vi "Change detector with tolerance threshold-DBL.vi"(6 "Tolerance (0.000001)":dbl=1e-06 format="%#_13f", 9 "From file":dbl[](array[numeric]), 11 "Current values":dbl[](array[numeric])) -> (2 "Changed?":bool[](array[boolean]))   [LabVIEW 2017]
panel:
  out "Difference":dbl[](array[numeric]) format="%#_6f"
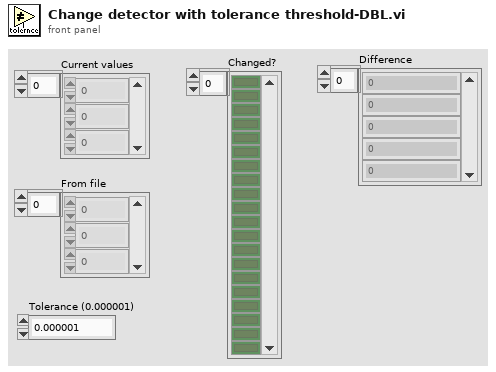
[diagram p1: front panel]
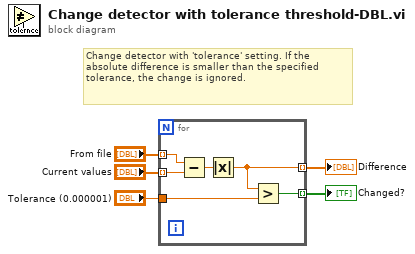
[diagram p0: block diagram]
diagram:
  # "Change detector with 'tolerance' setting. If the absolute difference is smaller than the specified tolerance, the change is ignored."
  n1 = for {
    tunnel: "From file" -> [w11] mode=indexing
    tunnel: "Current values" -> [w10] mode=indexing
    tunnel: [w6] -> w3 mode=indexing
    tunnel: [w8] -> w2 mode=indexing
    tunnel: "Tolerance (0.000001)" -> [w7]
    n2 = Subtract(x=w11, y=w10) -> (x-y=w9:dbl)
    n3 = Absolute Value(x=w9) -> (abs(x)=w6:dbl)
    n4 = Greater?(x=w6, y=w7) -> (0:w8:bool)
  }
  "Difference" <- w3
  "Changed?" <- w2
